vi "Write UniqueName.vi"(10 "Unique Name":string, 11 "Attribute.Identity in":refnum<class "Attribute.Identity.lvclass">) -> (3 "Attribute.Identity out":refnum<class "Attribute.Identity.lvclass">)   [LabVIEW 2021, in "smo.lvlib" / "Attribute.Identity.lvclass"]
uses:
  Attribute.Identity.lvclass
  Attribute.Identity.lvclass/Attribute.Identity.ctl
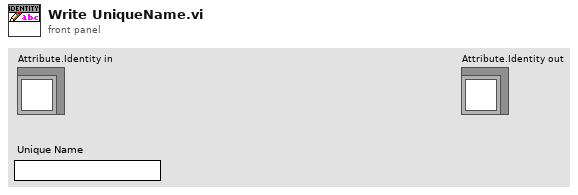
[diagram p1: front panel]
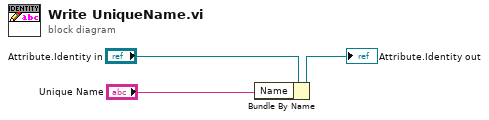
[diagram p0: block diagram]
diagram:
  n1 = Bundle By Name(cluster="Attribute.Identity in", "Name"="Unique Name") -> (→"Attribute.Identity out":refnum<class "Attribute.Identity.lvclass">)
